vi "Heater Main PID 2.vi"() -> ()   [LabVIEW 2019]
doc: "This example demonstrates how to acquire a continuous amount of data (Waveform) using the DAQ device's internal clock. It also shows how to synchronize two devices for different device families (E Series, S Series, M Series, X Series, DSA, and SC Express), to simultaneously acquire the data.\n\nFor instructions on how to connect your signals to the DAQ device, refer to your device documentation."
uses:
  <vilib>/Utility/error.llb/DialogType.ctl
  <vilib>/DAQmx/write.llb/DAQmx Write (Analog DBL 1Chan 1Samp).vi
  <vilib>/DAQmx/read.llb/DAQmx Read (Analog 1D Wfm NChan NSamp).vi
  <vilib>/DAQmx/configure/timing.llb/DAQmx Timing (Sample Clock).vi
  <vilib>/DAQmx/miscellaneous.llb/DAQmx Fill In Error Info.vi
panel:
  in  "Microhotplate Logger":T1(tab)=enum."Heater config"
  in  "Stop":bool
  in  "Enable logging":bool caption="Enable"
  in  "File config":T2={"Filepath"=path "C:/Users/Administrator/Desktop/DAQ Heater Control/Test data", "Test ID"="test", "PC"="69DTQV2"}
  in  "Sampling config":cluster{"Fs":dbl, "#s":dbl}={"Fs"=1000.0, "#s"=1000.0} {"Fs" format="%.2p"}
  out "Logging":bool
  in  "Output channel config":T3={"Output channel"="Dev1/ao0", "name to assign"="Heater Voltage"}
  in  "Voltage limit":dbl=3.0 caption="Amplitude"
  in  "Current channel config":T4={"Channel Index"=1, "Shunt resistance"=10.0, "Channel name"="Heater Current"} {"Shunt resistance" format="%.4f"}
  in  "IV channel config":T5={"Voltage channel index"=0, "Current channel index"=2}
  out "IV channel names":T6={"Voltage channel name"="Heater Voltage", "Current channel name"="Heater Current"}
  in  "TCR config":T7={"TCR1"=0.00205, "TCR2"=3e-07, "TRH"=0.766, "TRM"=0.928} {"TRM" format="%.3f"; "TRH" format="%.3f"; "TCR2" format="%.2e"; "TCR1" format="%.2e"}
  in  "Ramb config":cluster{"Tamb":dbl, "Ramb":dbl}={"Tamb"=25.0, "Ramb"=4.84} {"Ramb" format="%.3f"; "Tamb" format="%.3f"}
  out "Shunt channel name":string="Heater Shunt"
  out "PID output":dbl=1.0
  out "PID input":dbl
  in  "Setpoint":i32=2
  in  "Increment":dbl format="%.4f"
  out "Overrange":bool
  out "Heater shunt":dynamicdata(graph)=[{"t0"=timestamp(3680167673.7458043 s since 1904-01-01), "dt"=0.001, "Y"=[0.23414337637449473], "attributes"=variant("NI_ChannelName"=variant(string "Heater Voltage (DC Voltage)"), "NI_OriginalChannelName"=variant(string "Heater Voltage"), "NI_UnitDescription"=variant(string "Volts"))}, {"t0"=timestamp(3680167673.7458158 s since 1904-01-01), "dt"=0.001, "Y"=[0.4133136878458651], "attributes"=variant("NI_ChannelName"=variant(string "Heater Shunt (DC Voltage)"), "NI_OriginalChannelName"=variant(string "Heater Shunt"), "NI_UnitDescription"=variant(string "Volts"))}, {"t0"=timestamp(3680167673.7458158 s since 1904-01-01), "dt"=0.001, "Y"=[0.04133136878458673], "attributes"=variant("NI_ChannelName"=variant(string "Heater Current (DC Voltage)"), "NI_OriginalChannelName"=variant(string "Heater Current"), "NI_UnitDescription"=variant(string "A"))}, {"t0"=timestamp(3680167673.7458043 s since 1904-01-01), "dt"=0.001, "Y"=[5.665028733285053], "attributes"=variant("NI_ChannelName"=variant(string "Heater Resistance (DC Voltage)"), "NI_OriginalChannelName"=variant(string "Heater Resistance"), "NI_UnitDescription"=variant(string "Ohms"))}, {"t0"=timestamp(3680167673.7458043 s since 1904-01-01), "dt"=0.001, "Y"=[0.009677466447099818], "attributes"=variant("NI_ChannelName"=variant(string "Heater Power (DC Voltage)"), "NI_OriginalChannelName"=variant(string "Heater Power"), "NI_UnitDescription"=variant(string "Ohms"))}, {"t0"=timestamp(3680167673.7458043 s since 1904-01-01), "dt"=0.001, "Y"=[124.29416718343353], "attributes"=variant("NI_ChannelName"=variant(string "Heater Temp (DC Voltage)"), "NI_OriginalChannelName"=variant(string "Heater Temp"), "NI_UnitDescription"=variant(string "degC"))}]
  out "Heater temperature":dynamicdata(graph)=[{"t0"=timestamp(3680167673.7458043 s since 1904-01-01), "dt"=0.001, "Y"=[0.23414337637449473], "attributes"=variant("NI_ChannelName"=variant(string "Heater Voltage (DC Voltage)"), "NI_OriginalChannelName"=variant(string "Heater Voltage"), "NI_UnitDescription"=variant(string "Volts"))}, {"t0"=timestamp(3680167673.7458158 s since 1904-01-01), "dt"=0.001, "Y"=[0.4133136878458651], "attributes"=variant("NI_ChannelName"=variant(string "Heater Shunt (DC Voltage)"), "NI_OriginalChannelName"=variant(string "Heater Shunt"), "NI_UnitDescription"=variant(string "Volts"))}, {"t0"=timestamp(3680167673.7458158 s since 1904-01-01), "dt"=0.001, "Y"=[0.04133136878458673], "attributes"=variant("NI_ChannelName"=variant(string "Heater Current (DC Voltage)"), "NI_OriginalChannelName"=variant(string "Heater Current"), "NI_UnitDescription"=variant(string "A"))}, {"t0"=timestamp(3680167673.7458043 s since 1904-01-01), "dt"=0.001, "Y"=[5.665028733285053], "attributes"=variant("NI_ChannelName"=variant(string "Heater Resistance (DC Voltage)"), "NI_OriginalChannelName"=variant(string "Heater Resistance"), "NI_UnitDescription"=variant(string "Ohms"))}, {"t0"=timestamp(3680167673.7458043 s since 1904-01-01), "dt"=0.001, "Y"=[0.009677466447099818], "attributes"=variant("NI_ChannelName"=variant(string "Heater Power (DC Voltage)"), "NI_OriginalChannelName"=variant(string "Heater Power"), "NI_UnitDescription"=variant(string "Ohms"))}, {"t0"=timestamp(3680167673.7458043 s since 1904-01-01), "dt"=0.001, "Y"=[124.29416718343353], "attributes"=variant("NI_ChannelName"=variant(string "Heater Temp (DC Voltage)"), "NI_OriginalChannelName"=variant(string "Heater Temp"), "NI_UnitDescription"=variant(string "degC"))}]
  out "Heater current":dynamicdata(graph)=[{"t0"=timestamp(3680167673.7458043 s since 1904-01-01), "dt"=0.001, "Y"=[0.23414337637449473], "attributes"=variant("NI_ChannelName"=variant(string "Heater Voltage (DC Voltage)"), "NI_OriginalChannelName"=variant(string "Heater Voltage"), "NI_UnitDescription"=variant(string "Volts"))}, {"t0"=timestamp(3680167673.7458158 s since 1904-01-01), "dt"=0.001, "Y"=[0.4133136878458651], "attributes"=variant("NI_ChannelName"=variant(string "Heater Shunt (DC Voltage)"), "NI_OriginalChannelName"=variant(string "Heater Shunt"), "NI_UnitDescription"=variant(string "Volts"))}, {"t0"=timestamp(3680167673.7458158 s since 1904-01-01), "dt"=0.001, "Y"=[0.04133136878458673], "attributes"=variant("NI_ChannelName"=variant(string "Heater Current (DC Voltage)"), "NI_OriginalChannelName"=variant(string "Heater Current"), "NI_UnitDescription"=variant(string "A"))}, {"t0"=timestamp(3680167673.7458043 s since 1904-01-01), "dt"=0.001, "Y"=[5.665028733285053], "attributes"=variant("NI_ChannelName"=variant(string "Heater Resistance (DC Voltage)"), "NI_OriginalChannelName"=variant(string "Heater Resistance"), "NI_UnitDescription"=variant(string "Ohms"))}, {"t0"=timestamp(3680167673.7458043 s since 1904-01-01), "dt"=0.001, "Y"=[0.009677466447099818], "attributes"=variant("NI_ChannelName"=variant(string "Heater Power (DC Voltage)"), "NI_OriginalChannelName"=variant(string "Heater Power"), "NI_UnitDescription"=variant(string "Ohms"))}, {"t0"=timestamp(3680167673.7458043 s since 1904-01-01), "dt"=0.001, "Y"=[124.29416718343353], "attributes"=variant("NI_ChannelName"=variant(string "Heater Temp (DC Voltage)"), "NI_OriginalChannelName"=variant(string "Heater Temp"), "NI_UnitDescription"=variant(string "degC"))}]
  out "Heater voltage":dynamicdata(graph)=[{"t0"=timestamp(3680167673.7458043 s since 1904-01-01), "dt"=0.001, "Y"=[0.23414337637449473], "attributes"=variant("NI_ChannelName"=variant(string "Heater Voltage (DC Voltage)"), "NI_OriginalChannelName"=variant(string "Heater Voltage"), "NI_UnitDescription"=variant(string "Volts"))}, {"t0"=timestamp(3680167673.7458158 s since 1904-01-01), "dt"=0.001, "Y"=[0.4133136878458651], "attributes"=variant("NI_ChannelName"=variant(string "Heater Shunt (DC Voltage)"), "NI_OriginalChannelName"=variant(string "Heater Shunt"), "NI_UnitDescription"=variant(string "Volts"))}, {"t0"=timestamp(3680167673.7458158 s since 1904-01-01), "dt"=0.001, "Y"=[0.04133136878458673], "attributes"=variant("NI_ChannelName"=variant(string "Heater Current (DC Voltage)"), "NI_OriginalChannelName"=variant(string "Heater Current"), "NI_UnitDescription"=variant(string "A"))}, {"t0"=timestamp(3680167673.7458043 s since 1904-01-01), "dt"=0.001, "Y"=[5.665028733285053], "attributes"=variant("NI_ChannelName"=variant(string "Heater Resistance (DC Voltage)"), "NI_OriginalChannelName"=variant(string "Heater Resistance"), "NI_UnitDescription"=variant(string "Ohms"))}, {"t0"=timestamp(3680167673.7458043 s since 1904-01-01), "dt"=0.001, "Y"=[0.009677466447099818], "attributes"=variant("NI_ChannelName"=variant(string "Heater Power (DC Voltage)"), "NI_OriginalChannelName"=variant(string "Heater Power"), "NI_UnitDescription"=variant(string "Ohms"))}, {"t0"=timestamp(3680167673.7458043 s since 1904-01-01), "dt"=0.001, "Y"=[124.29416718343353], "attributes"=variant("NI_ChannelName"=variant(string "Heater Temp (DC Voltage)"), "NI_OriginalChannelName"=variant(string "Heater Temp"), "NI_UnitDescription"=variant(string "degC"))}]
  out "Heater resistance":dynamicdata(graph)=[{"t0"=timestamp(3680167673.7458043 s since 1904-01-01), "dt"=0.001, "Y"=[0.23414337637449473], "attributes"=variant("NI_ChannelName"=variant(string "Heater Voltage (DC Voltage)"), "NI_OriginalChannelName"=variant(string "Heater Voltage"), "NI_UnitDescription"=variant(string "Volts"))}, {"t0"=timestamp(3680167673.7458158 s since 1904-01-01), "dt"=0.001, "Y"=[0.4133136878458651], "attributes"=variant("NI_ChannelName"=variant(string "Heater Shunt (DC Voltage)"), "NI_OriginalChannelName"=variant(string "Heater Shunt"), "NI_UnitDescription"=variant(string "Volts"))}, {"t0"=timestamp(3680167673.7458158 s since 1904-01-01), "dt"=0.001, "Y"=[0.04133136878458673], "attributes"=variant("NI_ChannelName"=variant(string "Heater Current (DC Voltage)"), "NI_OriginalChannelName"=variant(string "Heater Current"), "NI_UnitDescription"=variant(string "A"))}, {"t0"=timestamp(3680167673.7458043 s since 1904-01-01), "dt"=0.001, "Y"=[5.665028733285053], "attributes"=variant("NI_ChannelName"=variant(string "Heater Resistance (DC Voltage)"), "NI_OriginalChannelName"=variant(string "Heater Resistance"), "NI_UnitDescription"=variant(string "Ohms"))}, {"t0"=timestamp(3680167673.7458043 s since 1904-01-01), "dt"=0.001, "Y"=[0.009677466447099818], "attributes"=variant("NI_ChannelName"=variant(string "Heater Power (DC Voltage)"), "NI_OriginalChannelName"=variant(string "Heater Power"), "NI_UnitDescription"=variant(string "Ohms"))}, {"t0"=timestamp(3680167673.7458043 s since 1904-01-01), "dt"=0.001, "Y"=[124.29416718343353], "attributes"=variant("NI_ChannelName"=variant(string "Heater Temp (DC Voltage)"), "NI_OriginalChannelName"=variant(string "Heater Temp"), "NI_UnitDescription"=variant(string "degC"))}]
  in  "Channel 2 config":T8={"Channel"="Dev1/ai3", "Vmax"=1.0, "Vmin"=0.0, "name to assign"="Heater Shunt", "input terminal configuration"=10106} {"input terminal configuration" items=["Default"=-1, "RSE"=10083, "NRSE"=10078, "Differential"=10106, "Pseudodifferential"=12529]; "Vmin" format="%0.2f"; "Vmax" format="%0.2f"}
  in  "Channel 1 config":T8={"Channel"="Dev1/ai2", "Vmax"=2.0, "Vmin"=0.0, "name to assign"="Heater Voltage", "input terminal configuration"=10106} {"input terminal configuration" items=["Default"=-1, "RSE"=10083, "NRSE"=10078, "Differential"=10106, "Pseudodifferential"=12529]; "Vmin" format="%0.2f"; "Vmax" format="%0.2f"}
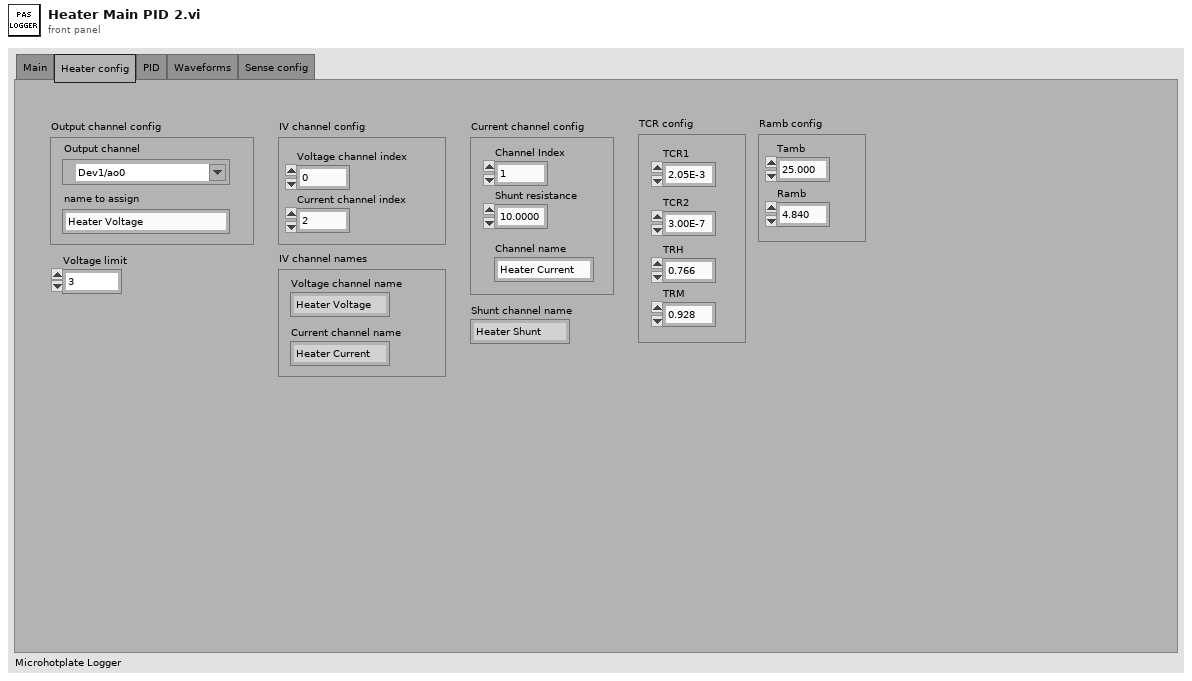
[diagram p1: front panel]
types:
  T1 = enum32{"Main", "Heater config", "PID", "Waveforms", "Sense config"}
  T2 = cluster{"Filepath":path, "Test ID":string, "PC":string}
  T3 = cluster{"Output channel":tag, "name to assign":string}
  T4 = cluster{"Channel Index":i32, "Shunt resistance":dbl, "Channel name":string}
  T5 = cluster{"Voltage channel index":i32, "Current channel index":i32}
  T6 = cluster{"Voltage channel name":string, "Current channel name":string}
  T7 = cluster{"TCR1":dbl, "TCR2":dbl, "TRH":dbl, "TRM":dbl}
  T8 = cluster{"Channel":tag, "Vmax":dbl, "Vmin":dbl, "name to assign":string, "input terminal configuration":i32}
  T9 = typedef "DialogType.ctl" = u16
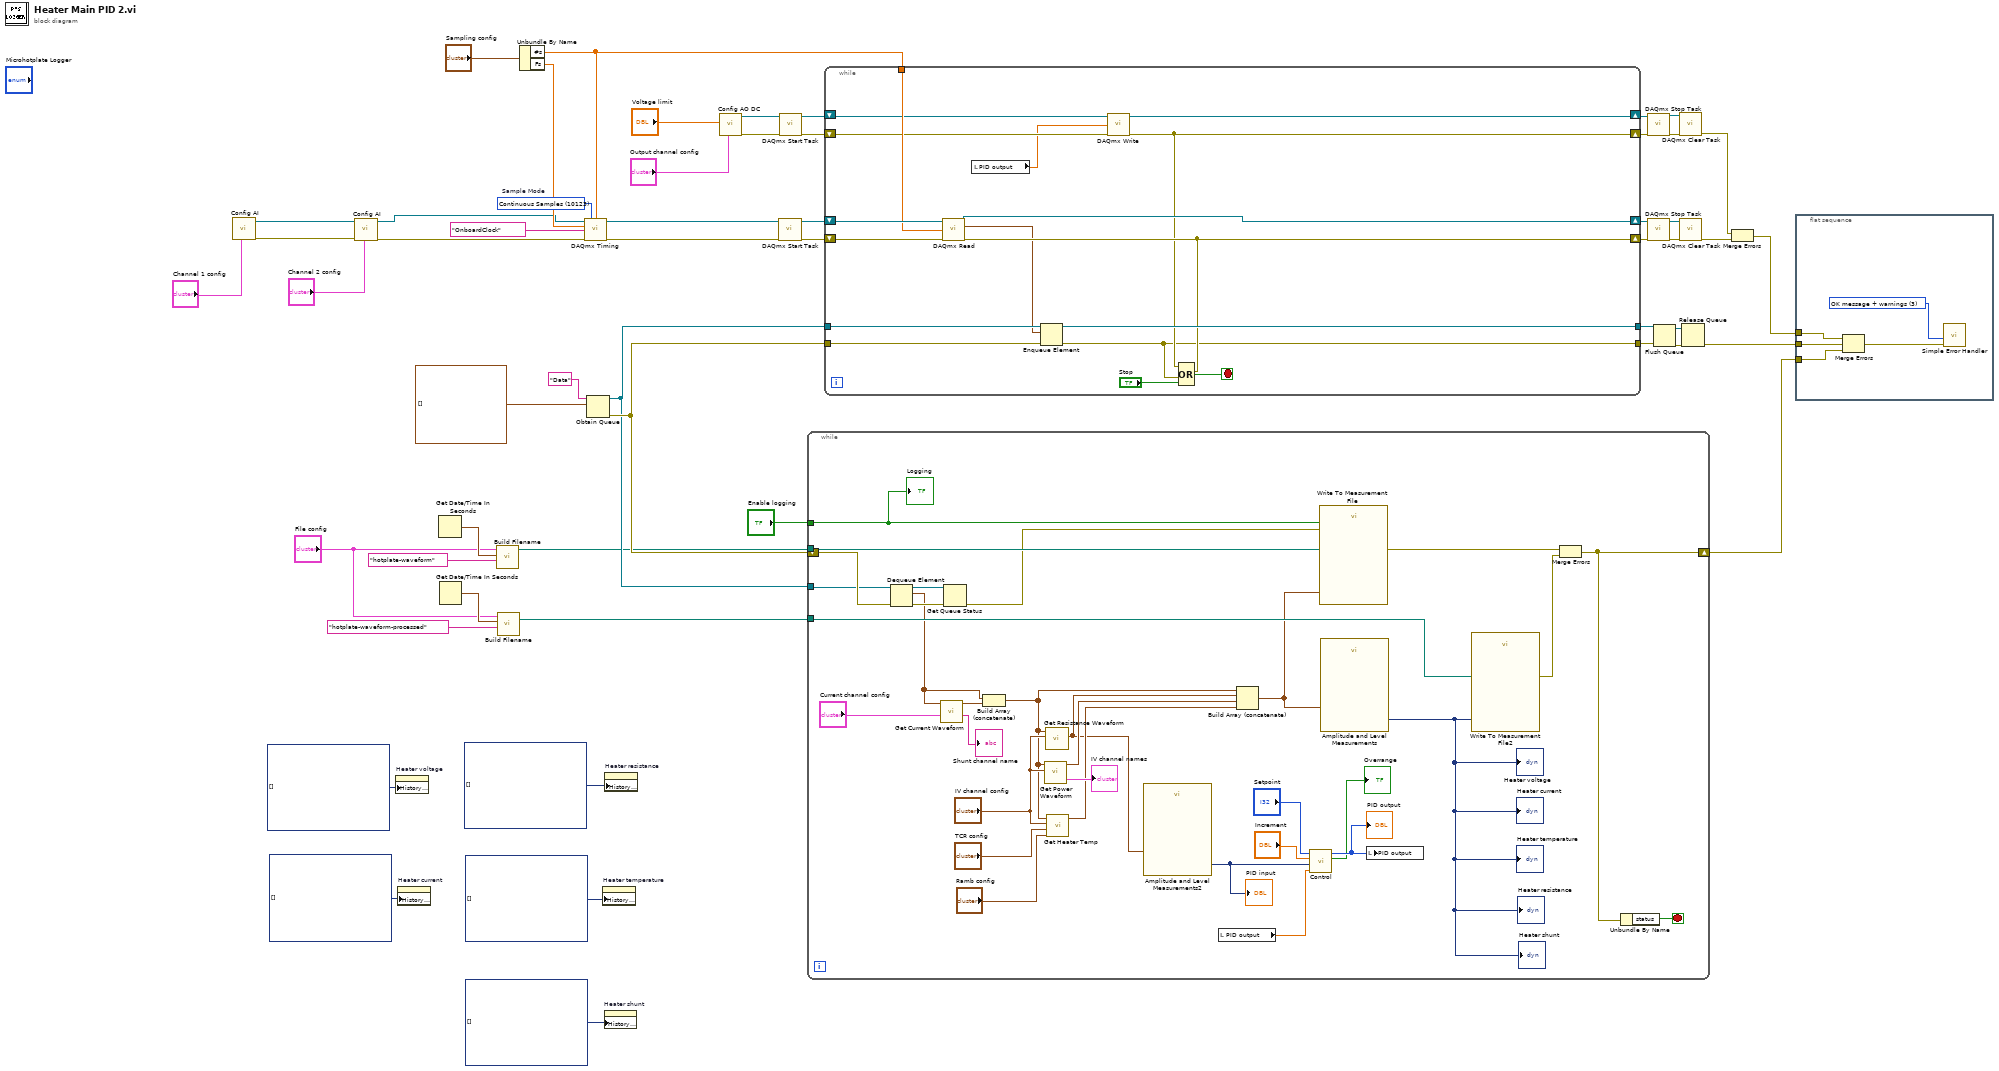
[diagram p0: block diagram]
diagram:
  w45 = 10123 items=["Finite Samples"=10178, "Continuous Samples"=10123, "Hardware Timed Single Point"=12522]  # Sample Mode
  n1 = call "Config AI.vi"("Channel config"="Channel 1 config") -> ("error out"=w26:errorcluster, "task out"=w25:refnum<k21>)  [unwired: 9 in]
  n2 = call "Config AI.vi"("Channel config"="Channel 2 config", "error in"=w26, "task in"=w25) -> ("error out"=w4:errorcluster, "task out"=w3:refnum<k21>)  [unwired: 7 in]
  n3 = property on="Heater voltage" class="WFChart (strict)"("History Data"=dynamicdata[] []) -> ()  [unwired: 2 in, 2 out]
  n4 = property on="Heater current" class="WFChart (strict)"("History Data"=dynamicdata[] []) -> ()  [unwired: 2 in, 2 out]
  n5 = Get Date/Time In Seconds() -> (seconds since 1Jan1904=w19:timestamp)
  n6 = Get Date/Time In Seconds() -> (seconds since 1Jan1904=w14:timestamp)
  n7 = call "Build Filename.vi"("Test type"="hotplate-waveform" ("File type"), "time stamp"=w19, "File config"="File config") -> ("appended path"=w21:path)  [unwired: 8 in]
  n8 = call "Build Filename.vi"("Test type"="hotplate-waveform-processed" ("File type"), "time stamp"=w14, "File config"="File config") -> ("appended path"=w13:path)  [unwired: 8 in]
  n9 = Unbundle By Name("Sampling config") -> ("#s"=w6:dbl, "Fs"=w5:dbl)
  n10 = call-poly <vilib>:"DAQmx Timing.vi"("task/channels in"=w3, "sample mode"=w45, "samples per channel"=w6, "rate"=w5, "source"=tag "OnboardClock", "error in"=w4) -> ("task out"=w11:refnum<k21>, "error out"=w10:errorcluster)  [unwired: 8 in]
  n11 = Obtain Queue(name (unnamed)="Data" ("名前（名前なし）"), element data type=waveform(dbl)[] [] ("data")) -> (queue out=w29:refnum<queue>, error out=w30:errorcluster)  [unwired: 3 in, 1 out]
  n12 = property on="Heater temperature" class="WFChart (strict)"("History Data"=dynamicdata[] []) -> ()  [unwired: 2 in, 2 out]
  n13 = property on="Heater shunt" class="WFChart (strict)"("History Data"=dynamicdata[] []) -> ()  [unwired: 2 in, 2 out]
  n14 = property on="Heater resistance" class="WFChart (strict)"("History Data"=dynamicdata[] []) -> ()  [unwired: 2 in, 2 out]
  n15 = call "Config AO DC.vi"("Channel config"="Output channel config", "Voltage"="Voltage limit") -> ("error out"=w39:errorcluster, "task out"=w40:refnum<k21>)  [unwired: 8 in]
  n16 = call <vilib>:"DAQmx Start Task.vi"("task/channels in"=w11, "error in"=w10) -> ("task out"=w41:refnum<k21>, "error out"=w42:errorcluster)  [unwired: 12 in]
  n17 = call <vilib>:"DAQmx Start Task.vi"("task/channels in"=w40, "error in"=w39) -> ("task out"=w43:refnum<k21>, "error out"=w44:errorcluster)  [unwired: 12 in]
  n18 = while {
    tunnel: w29 -> [w86]
    shift-right: [w79] -> w28
    shift-left: w30 -> [w87]
    tunnel: w21 -> [w85]
    tunnel: "Enable logging" -> [w81]
    tunnel: w13 -> [w76]
    stop <- w78 stop-if-true
    n19 = Dequeue Element(queue=w86, error in (no error)=w87) -> (queue out=w83:refnum<queue>, element=w67:waveform(dbl)[], error out=w84:errorcluster)  [unwired: 1 in, 1 out]
    n20 = call "Get Current Waveform.vi"("Config"="Current channel config", "array"=w67) -> ("Channel name"=→"Shunt channel name":string, "Current waveform out"=w73:waveform(dbl))  [unwired: 8 in]
    n21 = Get Queue Status(queue=w83, error in (no error)=w84) -> (error out=w82:errorcluster)  [unwired: 1 in, 7 out]
    n22 = Build Array (concatenate)(w67, w73) -> (w65:waveform(dbl)[])
    n23 = call "Get Power Waveform.vi"("Channel config"="IV channel config", "array"=w65) -> ("Power waveform out"=w68:waveform(dbl), "Channel names"=→"IV channel names":T6)  [unwired: 8 in]
    n24 = call "Get Resistance Waveform.vi"("Channel config"="IV channel config", "array"=w65) -> ("Resistance waveform out"=w58:waveform(dbl))  [unwired: 8 in, 1 out]
    n25 = call "Get Heater Temp.vi"("Ramb config"="Ramb config", "TCR config"="TCR config", "Channel config"="IV channel config", "array"=w65) -> ("waveform out"=w63:waveform(dbl))  [unwired: 6 in, 1 out]
    n26 = call "Amplitude and Level Measurements2"("Signals"=w58) -> ("Mean (DC)"=w57:dynamicdata)  [unwired: 13 in, 1 out]
    "PID input" <- w57
    n27 = local read "PID output"() -> (w59:dbl)
    n28 = Build Array (concatenate)(w65, w58, w68, w63) -> (w75:waveform(dbl)[])
    n29 = call "Control.vi"("Control in"=w59, "Sense"=w57, "Increment"="Increment", "Setpoint"="Setpoint") -> ("Overrange"=→"Overrange":bool, "Control out"=w60:i32)  [unwired: 6 in]
    "PID output" <- w60
    n30 = call "Write To Measurement File"("Signals"=w75, "Enable"=w81, "error in (no error)"=w82, "Filename"=w85) -> ("error out"=w80:errorcluster)  [unwired: 13 in, 2 out]
    n31 = call "Amplitude and Level Measurements"("Signals"=w75) -> ("Mean (DC)"=w66:dynamicdata)  [unwired: 13 in, 1 out]
    "Heater voltage" <- w66
    "Heater current" <- w66
    "Heater temperature" <- w66
    "Heater resistance" <- w66
    "Heater shunt" <- w66
    n32 = local write "PID output"(w60) -> ()
    n33 = call "Write To Measurement File2"("Signals"=w66, "Filename"=w76) -> ("error out"=w77:errorcluster)  [unwired: 15 in, 2 out]
    n34 = Merge Errors(w80, w77) -> (w79:errorcluster)
    n35 = Unbundle By Name(w79) -> ("status"=w78:bool)
    "Logging" <- w81
  }
  n36 = while {
    shift-right: [w92] -> w54
    shift-left: w44 -> [w93]
    shift-right: [w95] -> w50
    shift-left: w42 -> [w102]
    shift-right: [w90] -> w55
    shift-left: w43 -> [w91]
    shift-right: [w101] -> w51
    shift-left: w41 -> [w103]
    tunnel: w6 -> [w100]
    tunnel: [w99] -> w35
    tunnel: [w89] -> w34
    tunnel: w29 -> [w98]
    tunnel: w30 -> [w97]
    stop <- w104 stop-if-true
    n37 = call-poly <vilib>:"DAQmx Read.vi"("task/channels in"=w103, "number of samples per channel"=w100, "error in"=w102) -> ("task out"=w101:refnum<k21>, "data"=w94:waveform(dbl)[], "error out"=w95:errorcluster)  [unwired: 10 in]
    n38 = local read "PID output"() -> (w88:dbl)
    n39 = Enqueue Element(queue=w98, element=w94, error in (no error)=w97) -> (queue out=w99:refnum<queue>, error out=w89:errorcluster)  [unwired: 1 in, 1 out]
    n40 = call-poly <vilib>:"DAQmx Write.vi"("task/channels in"=w91, "data"=w88, "error in"=w93) -> ("task out"=w90:refnum<k21>, "error out"=w92:errorcluster)  [unwired: 10 in, 1 out]
    n41 = Compound Arithmetic op=OR(w92, w95, w89, "Stop") -> (w104:bool)
  }
  n42 = call <vilib>:"DAQmx Stop Task.vi"("task/channels in"=w55, "error in"=w54) -> ("task out"=w52:refnum<k21>, "error out"=w53:errorcluster)  [unwired: 12 in]
  n43 = call <vilib>:"DAQmx Stop Task.vi"("task/channels in"=w51, "error in"=w50) -> ("task out"=w48:refnum<k21>, "error out"=w49:errorcluster)  [unwired: 12 in]
  n44 = Flush Queue(queue=w35, error in (no error)=w34) -> (queue out=w36:refnum<queue>, error out=w37:errorcluster)  [unwired: 1 out]
  n45 = call <vilib>:"DAQmx Clear Task.vi"("task in"=w52, "error in"=w53) -> ("error out"=w47:errorcluster)  [unwired: 13 in]
  n46 = call <vilib>:"DAQmx Clear Task.vi"("task in"=w48, "error in"=w49) -> ("error out"=w46:errorcluster)  [unwired: 13 in]
  n47 = Release Queue(queue=w36, error in (no error)=w37) -> (error out=w32:errorcluster)  [unwired: 1 in, 2 out]
  n48 = Merge Errors(w47, w46) -> (w33:errorcluster)
  n49 = flat-sequence {
    tunnel: w33 -> [w109]
    tunnel: w32 -> [w108]
    tunnel: w28 -> [w105]
    frame #0 {
      w107 = T9 3 items=["no dialog", "OK message", "continue or stop message", "OK message + warnings", "continue/stop + warnings"] ("type of dialog (OK msg:1)")
      n50 = Merge Errors(w109, w108, w105) -> (w106:errorcluster)
      n51 = call <vilib>:"Simple Error Handler.vi"("type of dialog (OK msg:1)"=w107, "error in (no error)"=w106) -> ()  [unwired: 3 in, 5 out]
    }
  }
